vi "9.array-indexing-in-for-loop.vi"() -> ()   [LabVIEW 2010]
panel:
  out "Array 2":dbl[](array[numeric])
  out "Array":dbl[](array[numeric])
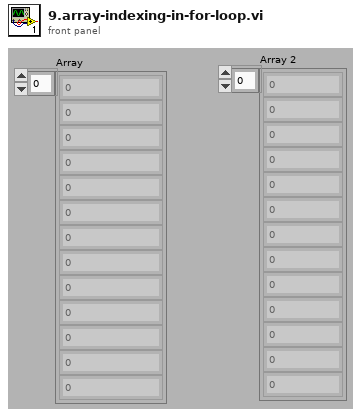
[diagram p1: front panel]
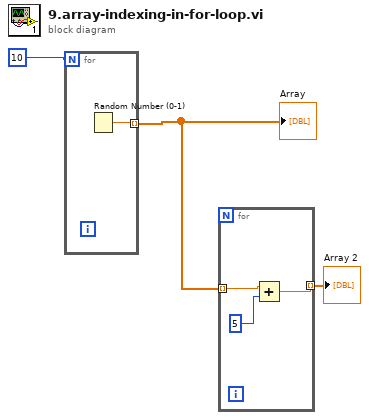
[diagram p0: block diagram]
diagram:
  n1 = for {
    N: 10 -> [_]
    tunnel: [w4] -> w2 mode=indexing
    n2 = Random Number (0-1)() -> (number: 0 to 1=w4:dbl)
  }
  "Array" <- w2
  n3 = for {
    tunnel: w2 -> [w7] mode=indexing
    tunnel: [w5] -> w1 mode=indexing
    n4 = Add(x=w7, y=5) -> (x+y=w5:dbl)
  }
  "Array 2" <- w1
